vi "SetWindowIcon.vi"(7 "Action":enum16{"Set", "Reset"}(ring), 8 "error in (no error)":errorcluster, 10 "VIRef (calling VI)":refnum<vi>, 11 "ICO Icon":path) -> (0 "Error Out":errorcluster)   [LabVIEW 2017]
doc: "Set a custom title bar icon for the referenced VI.\nIf no VI reference is supplied the VI calling this function is altered.\n\nUse <b>set</b> to change the icon to a custom icon, and <b>reset</b> to revert the icon to the previous value."
uses:
  C:/Windows/System32/user32.dll
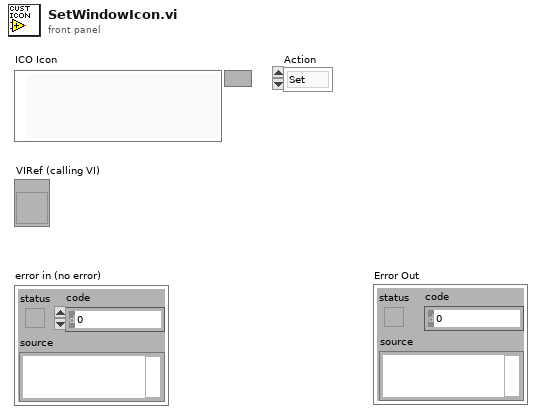
[diagram p1: front panel]
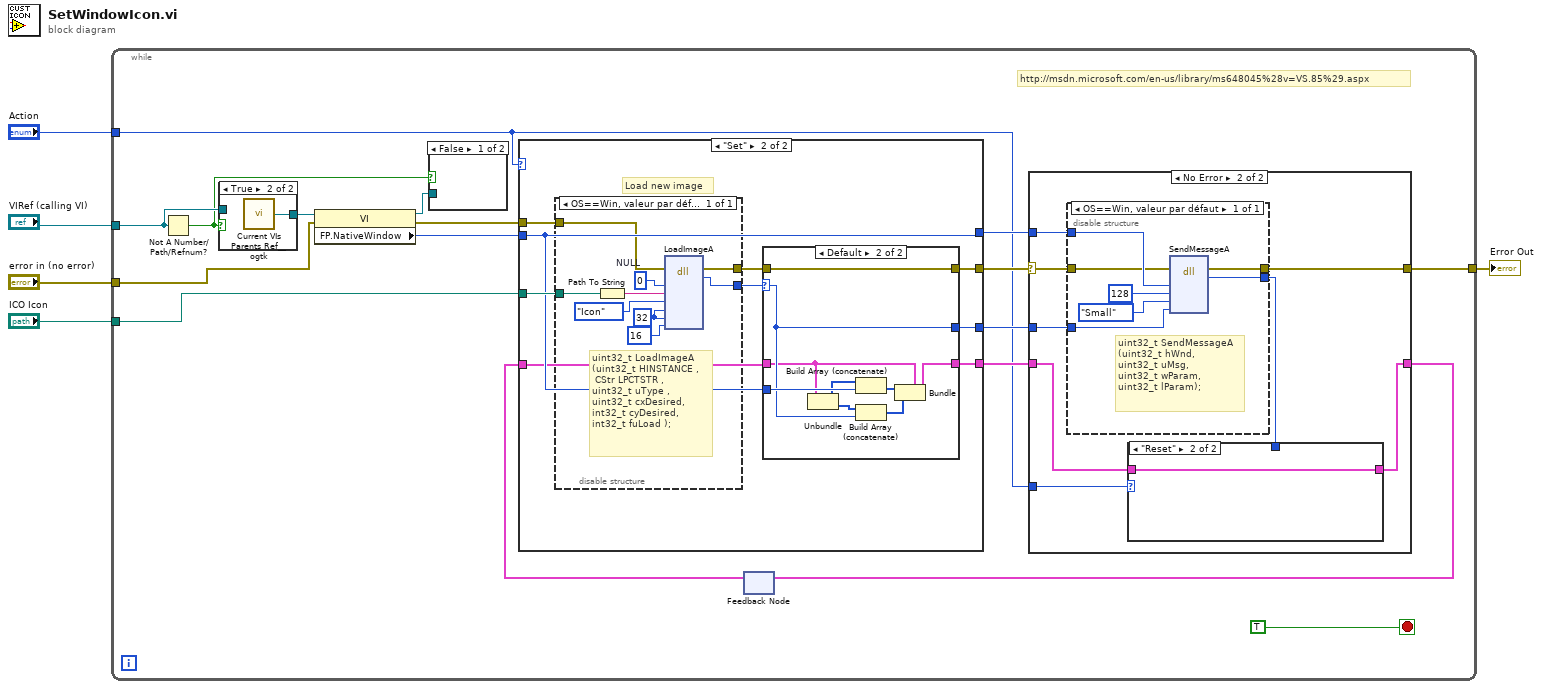
[diagram p0: block diagram]
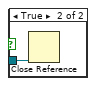
[diagram p2: hidden frame]
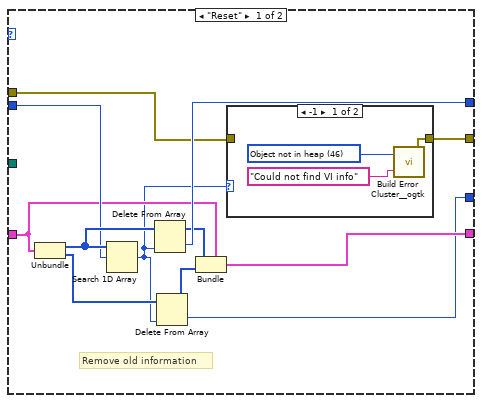
[diagram p3: hidden frame]
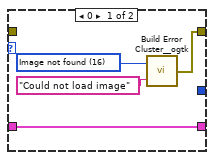
[diagram p5: hidden frame]
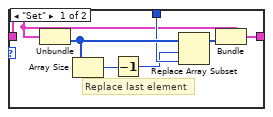
[diagram p8: hidden frame]
diagram:
  n1 = while {
    tunnel: "ICO Icon" -> [w22]
    tunnel: "error in (no error)" -> [w18]
    tunnel: "VIRef (calling VI)" -> [w21]
    tunnel: "Action" -> [w6]
    tunnel: [w11] -> w1
    stop <- TRUE stop-if-true
    # "http://msdn.microsoft.com/en-us/library/ms648045%28v=VS.85%29.aspx"
    n2 = Not A Number/Path/Refnum?(number/path/refnum=w21) -> (NaN/Path/Refnum?=w9:bool)
    n3 = case shown="True" w9 {
      tunnel: [w71 w72] -> w19
      tunnel: w21 -> [w71 _]
      frame False {
      }
      frame True {
        n4 = call <userlib>:"Current VIs Parents Ref__ogtk.vi"() -> ("Calling VI's Reference"=w72:refnum<vi>)  [unwired: 2 in]
      }
    }
    n5 = property class="VI"(reference=w19, error in=w18) -> (reference out=w10:refnum<vi>, error out=w17:errorcluster, "FP.NativeWindow"=w16:u64)
    n6 = case shown="False" w9 {
      tunnel: w10 -> [_ w23]
      frame False {
      }
      frame True {
        n7 = Close Reference(reference=w23) -> ()  [unwired: 1 in, 1 out]
      }
    }
    n8 = feedback #1() -> (w12:cluster{u64[], u32[]})  [unwired: 1 in]
    n9 = case shown="\"Set\"" w6 {
      tunnel: w22 -> [_ w48]
      tunnel: [w24 w44] -> w14
      tunnel: [w27 w45] -> w13
      tunnel: w17 -> [w25 w47]
      tunnel: [w33 w42] -> w15
      tunnel: w16 -> [w34 w42]
      tunnel: w12 -> [w29 w41]
      tunnel: [w28 w40] -> w8
      frame "Reset" {
        # "Remove old information"
        n10 = Unbundle(w29) -> (w35:u64[], w32:u32[])
        n11 = Search 1D Array(1D array=w35, element=w34) -> (index of element=w26:i32)  [unwired: 1 in]
        n12 = Delete From Array(array=w35, index=w26) -> (deleted portion=w33:u64, array with subset deleted=w31:u64[])  [unwired: 1 in]
        n13 = Delete From Array(array=w32, index=w26) -> (deleted portion=w27:u32, array with subset deleted=w30:u32[])  [unwired: 1 in]
        n14 = Bundle(cluster=w29, w31, w30) -> (w28:cluster{u64[], u32[]})
        n15 = case shown="-1" w26 {
          tunnel: [w36 w39] -> w24
          tunnel: w25 -> [_ w39]
          frame -1 {
            w37 = 46 items=["No error", "Argument error", "Memory is full", "Out of zone", "End of file", "File already open", "Generic file I/O error", "File not found", "File permission error", "Disk is full", "Duplicate path", "Too many files open", "System feature not enabled", "Resource file not found", "Cannot add resource", "Resource not found", "Image not found", "Image memory error", "Pen does not exist", "Config type invalid", "Config token not found", "Config parse error", "Config memory error", "Bad external code format", "Bad external code offset", "External code not present", "Null window", "Destroy window error", "Null menu", "Print aborted", "Bad print record", "Print driver error", "Windows error during printing", "Memory error during printing", "Print dialog error", "Generic print error", "Invalid device refnum", "Device not found", "Device parameter error", "Device unit error", "Cannot open device", "Device call aborted", "Generic error", "Cancelled by user", "Object ID too low", "Object ID too high", "Object not in heap", "Unknown heap", "Unknown object (invalid DefProc)", "Unknown object (DefProc not in table)", "Message out of range", "Invalid (null) method", "Unknown message", "Manager call not supported", "Bad address", "Network operation in progress", "Network operation timed out", "Connection is busy", "Network attribute not supported", "Network error", "Address in use", "System out of memory", "Connection aborted", "Connection refused", "Not connected", "Already connected", "Connection closed", "Initialization error (interapplication manager)", "Bad occurrence", "Wait on unbound occurrence handler", "Occurrence queue overflow", "Datalog type conflict", "Unused", "Unrecognized type (interapplication manager)", "Memory corrupt", "Failed to make temporary DLL", "Old CIN version", "Drag socket not found", "Failed to load drop-object", "Failed to register OLE object", "Failed to release OLE object", "Format specifier type mismatch", "Unknown format specifier", "Too few format specifiers", "Too many format specifiers", "Scan failed", "Newer CIN version", "Error converting to variant", "Runtime menu error", "Password tampered", "Variant attribute not found", "Incompatible variant data type", "Event data is not available", "Event Store is not present", "Occurrence is not found", "Event Queue is not created", "Event info is not available", "Refnum passed is NULL", "Error retrieving Class GUID", "Error retrieving CoClass GUID", "Error retrieving TypeLib GUID.", "Bad built application magic bytes.", "Specific driver is different from the specific driver associated with the Logical Name.", "There is no session opened to the class driver.", "Max Error", "MAX - Error with config objects", "MAX - Error loading configuration", "MAX - Group not supported"]
            n16 = call <userlib>:"Build Error Cluster__ogtk.vi"("String to Prepend to source (\"\")"="Could not find VI info" ("source"), "code"=w37) -> ("error out"=w36:errorcluster)
          }
          frame Default {
          }
        }
      }
      frame "Set" {
        # "Load new image"
        n17 = disable-structure shown="OS==Win, valeur par défaut" {
          disable-tunnel: w48 -> [w54]
          disable-tunnel: w47 -> [w52]
          disable-tunnel: [w50] -> w46
          disable-tunnel: [w49] -> w43
          frame condition #0 (active) {
            w56 = u32 32 ("cxDesired")
            w57 = u32 0  # NULL
            # "uint32_t LoadImageA\n(uint32_t HINSTANCE ,\n CStr LPCTSTR ,\nuint32_t uType , \nuint32_t cxDesired, \nint32_t cyDesired, \nint32_t fuLoad );"
            n18 = Path To String(path=w54) -> (string=w53:string)
            n19 = dll-call lib="C:/Windows/System32/user32.dll" fn="LoadImageA" label="LoadImage"(error in=w52, "HINSTANCE"=w57, "LPCTSTR"=w53, "uType"=enum16{"Bitmap", "Icon", "Cursor"}."Icon", "cxDesired"=w56, "cyDesired"=w56, "fuLoad"=16) -> (error out=w49:errorcluster, "ImageHandle"=w50:u32)  [unwired: 8 in, 1 out]
          }
        }
        n20 = case shown="Default" w46 {
          selector: w46 -> [_ w68]
          tunnel: [_ w68] -> w45
          tunnel: [w58 w70] -> w44
          tunnel: w43 -> [_ w70]
          tunnel: w42 -> [_ w69]
          tunnel: w41 -> [w61 w64]
          tunnel: [w61 w65] -> w40
          frame 0 {
            w60 = 16 items=["No error", "Argument error", "Memory is full", "Out of zone", "End of file", "File already open", "Generic file I/O error", "File not found", "File permission error", "Disk is full", "Duplicate path", "Too many files open", "System feature not enabled", "Resource file not found", "Cannot add resource", "Resource not found", "Image not found", "Image memory error", "Pen does not exist", "Config type invalid", "Config token not found", "Config parse error", "Config memory error", "Bad external code format", "Bad external code offset", "External code not present", "Null window", "Destroy window error", "Null menu", "Print aborted", "Bad print record", "Print driver error", "Windows error during printing", "Memory error during printing", "Print dialog error", "Generic print error", "Invalid device refnum", "Device not found", "Device parameter error", "Device unit error", "Cannot open device", "Device call aborted", "Generic error", "Cancelled by user", "Object ID too low", "Object ID too high", "Object not in heap", "Unknown heap", "Unknown object (invalid DefProc)", "Unknown object (DefProc not in table)", "Message out of range", "Invalid (null) method", "Unknown message", "Manager call not supported", "Bad address", "Network operation in progress", "Network operation timed out", "Connection is busy", "Network attribute not supported", "Network error", "Address in use", "System out of memory", "Connection aborted", "Connection refused", "Not connected", "Already connected", "Connection closed", "Initialization error (interapplication manager)", "Bad occurrence", "Wait on unbound occurrence handler", "Occurrence queue overflow", "Datalog type conflict", "Unused", "Unrecognized type (interapplication manager)", "Memory corrupt", "Failed to make temporary DLL", "Old CIN version", "Drag socket not found", "Failed to load drop-object", "Failed to register OLE object", "Failed to release OLE object", "Format specifier type mismatch", "Unknown format specifier", "Too few format specifiers", "Too many format specifiers", "Scan failed", "Newer CIN version", "Error converting to variant", "Runtime menu error", "Password tampered", "Variant attribute not found", "Incompatible variant data type", "Event data is not available", "Event Store is not present", "Occurrence is not found", "Event Queue is not created", "Event info is not available", "Refnum passed is NULL", "Error retrieving Class GUID", "Error retrieving CoClass GUID", "Error retrieving TypeLib GUID.", "Bad built application magic bytes.", "Specific driver is different from the specific driver associated with the Logical Name.", "There is no session opened to the class driver.", "Max Error", "MAX - Error with config objects", "MAX - Error loading configuration", "MAX - Group not supported"]
            n21 = call <userlib>:"Build Error Cluster__ogtk.vi"("String to Prepend to source (\"\")"="Could not load image" ("source"), "code"=w60) -> ("error out"=w58:errorcluster)
          }
          frame Default {
            n22 = Unbundle(w64) -> (w63:u64[], w62:u32[])
            n23 = Build Array (concatenate)(w63, w69) -> (w67:u64[])
            n24 = Build Array (concatenate)(w62, w68) -> (w66:u32[])
            n25 = Bundle(cluster=w64, w67, w66) -> (w65:cluster{u64[], u32[]})
          }
        }
      }
    }
    n26 = case shown="No Error" w14 {
      selector: w14 -> [w74 w79]
      tunnel: [w74 w82] -> w11
      tunnel: w15 -> [_ w81]
      tunnel: w13 -> [_ w80]
      tunnel: w8 -> [w73 w76]
      tunnel: [w73 w77] -> w7
      tunnel: w6 -> [_ w75]
      frame Error {
      }
      frame No Error {
        n27 = disable-structure shown="OS==Win, valeur par défaut" {
          disable-tunnel: [w97] -> w82
          disable-tunnel: w81 -> [w95]
          disable-tunnel: w80 -> [w93]
          disable-tunnel: w79 -> [w92]
          disable-tunnel: [w91] -> w78
          frame condition #0 (active) {
            # "uint32_t SendMessageA\n(uint32_t hWnd,\nuint32_t uMsg,\nuint32_t wParam,\nuint32_t lParam);"
            n28 = dll-call lib="C:/Windows/System32/user32.dll" fn="SendMessageA" label="SendMessage"(error in=w92, "hWnd"=w95, "uMsg"=128 ("dimension size"), "wParam"=enum16{"Small", "Big"}."Small", "lParam"=w93) -> (error out=w97:errorcluster, "OldHandle"=w91:u32)  [unwired: 6 in, 1 out]
          }
        }
        n29 = case shown="\"Reset\"" w75 {
          tunnel: w78 -> [w88 _]
          tunnel: [w84 w90] -> w77
          tunnel: w76 -> [w83 w90]
          frame "Set" {
            # "Replace last element"
            n30 = Unbundle(w83) -> (w89:u32[])  [unwired: 1 out]
            n31 = Array Size(array=w89) -> (size(s)=w87:i32)
            n32 = Decrement(x=w87) -> (x-1=w86:i32)
            n33 = Replace Array Subset(array=w89, new element=w88, index=w86) -> (w85:u32[])
            n34 = Bundle(cluster=w83, w85) -> (w84:cluster{u64[], u32[]})  [unwired: 1 in]
          }
          frame "Reset" {
          }
        }
      }
    }
    n35 = feedback-in #1(w7) -> ()
  }
  "Error Out" <- w1
